vi "5.vi"   [LabVIEW 2017]
types:
  T1 = enum16{"open", "replace", "create", "open or create", "replace or create", "replace or create with confirmation"}
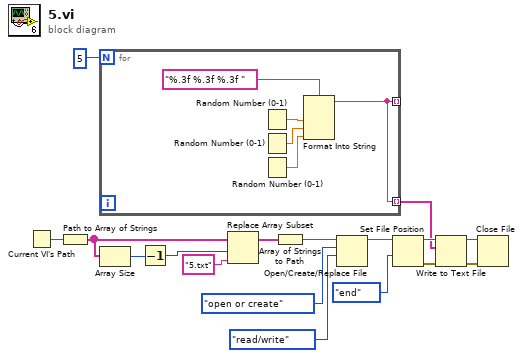
[diagram p0: block diagram]
diagram:
  n1 = Current VI's Path() -> (path=w7:path)
  n2 = Path to Array of Strings(0:w7) -> (2:w6:string[])  [unwired: 1 out]
  n3 = for {
    N: 5 -> [_]
    tunnel: [w18] -> _ mode=indexing
    tunnel: [w18] -> w8 mode=indexing
    n4 = Random Number (0-1)() -> (number: 0 to 1=w22:dbl)
    n5 = Random Number (0-1)() -> (number: 0 to 1=w20:dbl)
    n6 = Random Number (0-1)() -> (number: 0 to 1=w19:dbl)
    n7 = Format Into String(format string="%.3f %.3f %.3f " ("初始字符串"), w22, w20, w19) -> (resulting string=w18:string)  [unwired: 2 in, 1 out]
  }
  n8 = Array Size(array=w6) -> (size(s)=w2:i32)
  n9 = Decrement(x=w2) -> (x-1=w1:i32)
  n10 = Replace Array Subset(array=w6, new element="5.txt" ("新元素/子数组"), index=w1) -> (w4:string[])
  n11 = Array of Strings to Path(0:w4) -> (2:w3:path)  [unwired: 1 in]
  n12 = Open/Create/Replace File(file path (use dialog)=w3, operation (0:open)=T1."open or create" ("操作(0:open)"), access (0:read/write)=enum16{"read/write", "read-only", "write-only"}."read/write" ("权限(0:read/write)")) -> (refnum out=w17:refnum<file>)  [unwired: 3 in, 2 out]
  n13 = Set File Position(refnum=w17, from (0:start)=enum16{"start", "end", "current"}."end" ("自（0:起始）")) -> (refnum out=w15:refnum<file>, error out=w14:errorcluster)  [unwired: 2 in]
  n14 = Write to Text File(file (use dialog)=w15, text=w8, error in=w14) -> (refnum out=w13:refnum<file>, error out=w12:errorcluster)  [unwired: 1 in, 1 out]
  n15 = Close File(refnum=w13, error in=w12) -> ()  [unwired: 2 out]
